vi "sv_Continuous Swept-Sine Tags.vi"(1 "chirp sweep tag selector":T1) -> (0 "Tag":string)   [LabVIEW 2017, in "SoundVib_ContSweptSine.lvlib"]
uses:
  <vilib>/addons/Sound and Vibration/svt_Continuous Swept Sine/SoundVib_ContSweptSine.lvlib
  <vilib>/addons/Sound and Vibration/svt_Continuous Swept Sine/subVIs/sv_Continuous Swept-Sine Tags.ctl
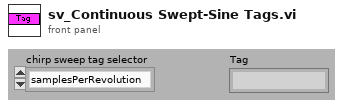
[diagram p1: front panel]
types:
  T1 = typedef "SoundVib_ContSweptSine.lvlib/sv_Continuous Swept-Sine Tags.ctl" = enum16{"samplesPerRevolution", "t2aPositions", "a2tPositions", "evenAngleSignal", "evenAnglePositionInfo", "evenAngleChannelInfo"}
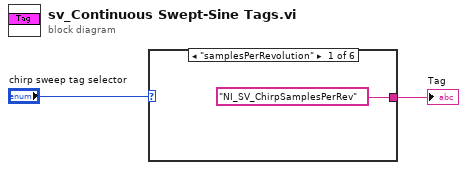
[diagram p0: block diagram]
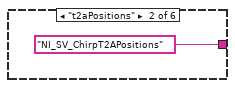
[diagram p2: hidden frame]
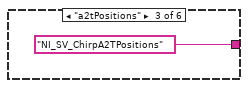
[diagram p3: hidden frame]
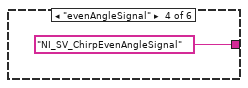
[diagram p4: hidden frame]
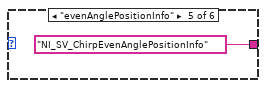
[diagram p5: hidden frame]
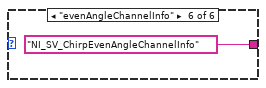
[diagram p6: hidden frame]
diagram:
  n1 = case shown="\"samplesPerRevolution\"" "chirp sweep tag selector" {
    tunnel: ["NI_SV_ChirpSamplesPerRev" "NI_SV_ChirpT2APositions" "NI_SV_ChirpA2TPositions" "NI_SV_ChirpEvenAngleSignal" "NI_SV_ChirpEvenAnglePositionInfo" "NI_SV_ChirpEvenAngleChannelInfo"] -> w1
    frame "samplesPerRevolution" {
    }
    frame "t2aPositions" {
    }
    frame "a2tPositions" {
    }
    frame "evenAngleSignal" {
    }
    frame "evenAnglePositionInfo" {
    }
    frame "evenAngleChannelInfo" {
    }
  }
  "Tag" <- w1
